vi "Pre Launch Init.vi"(11 "He Line in":refnum<class "He Line.lvclass">) -> (0 "error out":errorcluster, 3 "He Line out":refnum<class "He Line.lvclass">)   [LabVIEW 2015, in "cRIO-Carbondioxide.lvlib" / "CO2-Actor.lvlib" / "He Line.lvclass"]
doc: "(<B>Filename</B>: Actor Framework.lvlib:Actor.lvclass:Pre Launch Init.vi)\n\nDefines behavior that occurs after the Launch Actor method is invoked but before the actor's Actor Core method begins running.\n\nThe Pre Launch Init method is guaranteed to finish before the Launch Actor method returns to its caller and before the actor itself receives any messages. Any references that the Pre Launch Init method obtains are guaranteed to have the same lifetime as the actor itself. Any errors that the Pre Launch Init method returns will abort the launch.\n\nBy default, this method does nothing. A descendant class may override it to define behavior."
uses:
  He Line.lvclass
  subs/Sample/Sample.lvclass
  He Line.lvclass/He Line.ctl
  Valve/Valve.lvclass
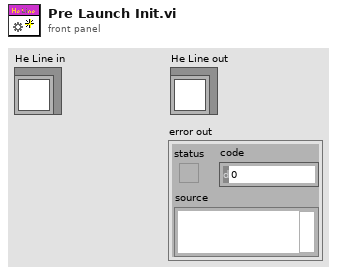
[diagram p1: front panel]
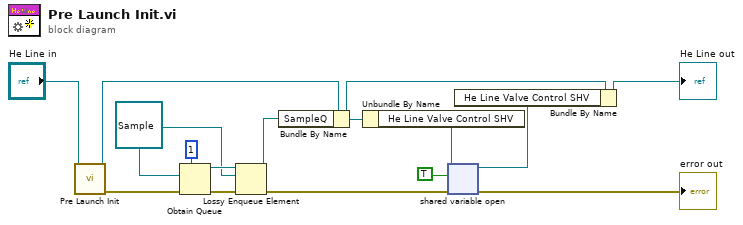
[diagram p0: block diagram]
diagram:
  w8 = refnum<class "Sample.lvclass"> refnum ("element")
  n1 = call-parent "Pre Launch Init.vi"("Valve in"="He Line in") -> ("error out"=w13:errorcluster, "Valve out"=w14:refnum<class "He Line.lvclass">)  [unwired: 9 in]
  n2 = Obtain Queue(max queue size (-1, unlimited)=1, element data type=w8, error in (no error)=w13) -> (queue out=w10:refnum<queue>, error out=w11:errorcluster)  [unwired: 2 in, 1 out]
  n3 = Lossy Enqueue Element(queue=w10, element=w8, error in (no error)=w11) -> (queue out=w9:refnum<queue>, error out=w6:errorcluster)  [unwired: 2 out]
  n4 = Bundle By Name(cluster=w14, "SampleQ"=w9) -> (w7:refnum<class "He Line.lvclass">)
  n5 = Unbundle By Name(w7) -> ("He Line Valve Control SHV"=w4:refnum<k21>)
  n6 = shared-variable-open(w4, w6, TRUE) -> (w1:refnum<k21>, →"error out":errorcluster)  [unwired: 1 in]
  n7 = Bundle By Name(cluster=w7, "He Line Valve Control SHV"=w1) -> (→"He Line out":refnum<class "He Line.lvclass">)
